vi "Error Handler - Message Handling Loop.vi"(8 "error in (no error)":errorcluster, 10 "Ignore Errors (Runtime)":i32[](array[numeric]), 11 "Message Queue":refnum<queue>) -> (0 "dup error in":errorcluster, 3 "dup Message Queue":refnum<queue>)   [LabVIEW 2019]
doc: "Process an error that occurred in the Message Handling Loop, either by ignoring it, or generating an \"Exit\" message."
uses:
  Message Cluster.ctl
  Message Queue.lvlib
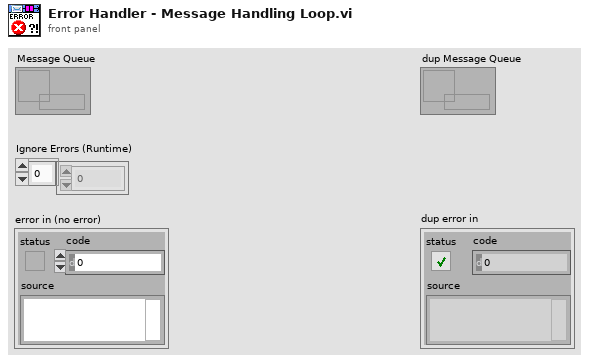
[diagram p1: front panel]
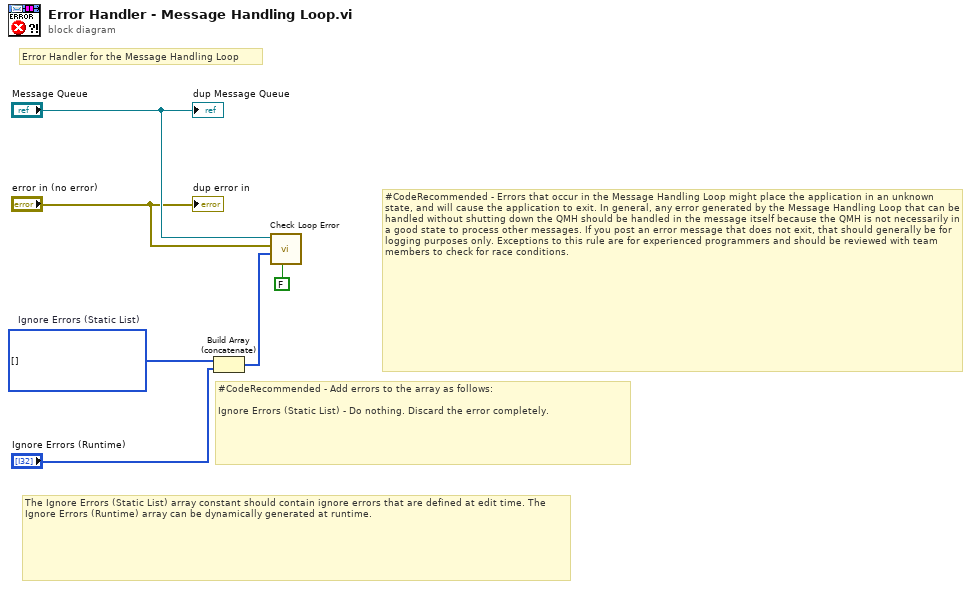
[diagram p0: block diagram]
diagram:
  w5 = i32[] []  # Ignore Errors (Static List)
  # "#CodeRecommended - Errors that occur in the Message Handling Loop might place the application in an unknown state, and will cause the application to exit. In general, any error generated by the Message Handling Loop that can be handled without shutting down the QMH should be handled in the message itself because the QMH is not necessarily in a good state to process other messages. If you post an error message that does not exit, that should generally be for logging purposes only. Exceptions to this rule are for experienced programmers and should be reviewed with team members to check for race conditions."
  # "The Ignore Errors (Static List) array constant should contain ignore errors that are defined at edit time. The Ignore Errors (Runtime) array can be dynamically generated at runtime."
  # "#CodeRecommended - Add errors to the array as follows:\n\nIgnore Errors (Static List) - Do nothing. Discard the error completely."
  # "Error Handler for the Message Handling Loop"
  n1 = Build Array (concatenate)(w5, "Ignore Errors (Runtime)") -> (w4:i32[])
  n2 = call "Check Loop Error.vi"("Exit on Error? (F)"=FALSE, "Ignore Errors"=w4, "error to process"="error in (no error)", "Message Queue"="Message Queue") -> ()  [unwired: 6 in, 2 out]
  "dup Message Queue" <- "Message Queue"
  "dup error in" <- "error in (no error)"
